vi "Main.vi"(11 "Module Admin":refnum<class "Delacor_lib_QMH_Cloneable Module Admin.lvclass">) -> ()   [LabVIEW 2024, in "CloneableSubpanel.lvlib"]
doc: "This template is based off of the Queued Message Handler design pattern and the Queued Message Handler project template that ships with LabVIEW.\n\nThe main difference is that the queue is private to this module and communication between modules is performed via Broadcast and Request events.\n\nRequest events are wrapped in public API methods and are handled in the Event Handling Loop (EHL) of this VI. Any module can register for Broadcast events sent by this module. The EHL generates messages based on user interface actions.\n\nThe Message Handling Loop (MHL) processes messages generated by the EHL, or by other messages. The messages are string values, so new messages can be added easily to the Message Cases case structure in the MHL. Each message cluster can also provide an optional value for Message Data, which is a variant that can be converted to whatever message-specific data is required.\n_____\nBased on DQMH Dev Tools: Project Template 7.1.0.1503."
uses:
  CloneableSubpanel.lvlib
  <vilib>/Delacor/Delacor QMH/Libraries/Cloneable Module Admin_class/Delacor_lib_QMH_Cloneable Module Admin.lvclass
  C:/Program Files (x86)/National Instruments/LabVIEW 2024/vi.lib/Delacor/Delacor QMH/Libraries/Module Admin_class/Delacor_lib_QMH_Module Admin.lvclass
  Module Data--cluster.ctl
  <vilib>/Delacor/Delacor QMH/Libraries/Message Queue_class/Delacor_lib_QMH_Message Queue.lvclass/Delacor_lib_QMH_Message Queue.ctl
  <vilib>/Delacor/Delacor QMH/Libraries/Cloneable Module Admin_class/Delacor_lib_QMH_Cloneable Module Admin.lvclass/Delacor_lib_QMH_Cloneable Module Admin.ctl
  Stop Argument--cluster.ctl
  <vilib>/Delacor/Delacor QMH/Libraries/Module Admin_class/Delacor_lib_QMH_Module Admin.lvclass/Delacor_lib_QMH_Module Admin.ctl
  Draw FP in Subpanel Argument--cluster.ctl
  Remove From Subpanel Argument--cluster.ctl
  <vilib>/Utility/miscctls.llb/LVPointTypeDef.ctl
  <vilib>/Delacor/Delacor QMH/Libraries/Message Queue_class/Delacor_lib_QMH_Enqueue Message (Single).vi
  <vilib>/Delacor/Delacor QMH/Libraries/Cloneable Module Admin_class/Delacor_lib_QMH_Get Module ID.vi
  <vilib>/Delacor/Delacor QMH/Libraries/Module Admin_class/Delacor_lib_QMH_Get External Launch.vi
  <vilib>/Delacor/Delacor QMH/Libraries/Message Queue_class/Delacor_lib_QMH_Message Queue.lvclass
panel:
  out "error out":errorcluster
  out "Status":string
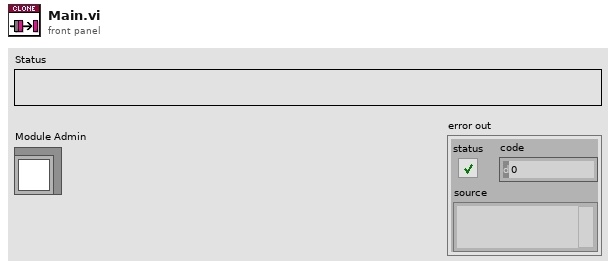
[diagram p1: front panel]
types:
  T1 = typedef "CloneableSubpanel.lvlib/Request Events--cluster.ctl" = cluster{"Stop Module":refnum<user-event>, "Show Panel":refnum<user-event>, "Hide Panel":refnum<user-event>, "Show Diagram":refnum<user-event>, "Get Module Execution Status":refnum<user-event>, "Draw FP in Subpanel":refnum<user-event>, "Remove From Subpanel":refnum<user-event>}
  T2 = typedef "CloneableSubpanel.lvlib/Module Data--cluster.ctl" = cluster{"Status":string, "Sub Panel":refnum<vi>}
  T3 = enum32{"invalid lock state", "Not Locked", "Locked (No Password)", "Password-protected"}
  T4 = typedef "CloneableSubpanel.lvlib/Stop Argument--cluster.ctl" = cluster{"Module ID":i32, "Origin":string, "Exit via Stop Module Req?":bool, "Wait for Module to stop?":bool}
  T5 = typedef "CloneableSubpanel.lvlib/Draw FP in Subpanel Argument--cluster.ctl" = cluster{"Module ID":i32, "Sub Panel":refnum<vi>}
  T6 = typedef "CloneableSubpanel.lvlib/Remove From Subpanel Argument--cluster.ctl" = cluster{"Module ID":i32, "Boolean":bool}
  T7 = typedef "LVPointTypeDef.ctl" = cluster{"Horizontal":i16, "Vertical":i16}
  T8 = enum32{"Invalid", "Standard", "Closed", "Hidden", "Minimized", "Maximized"}
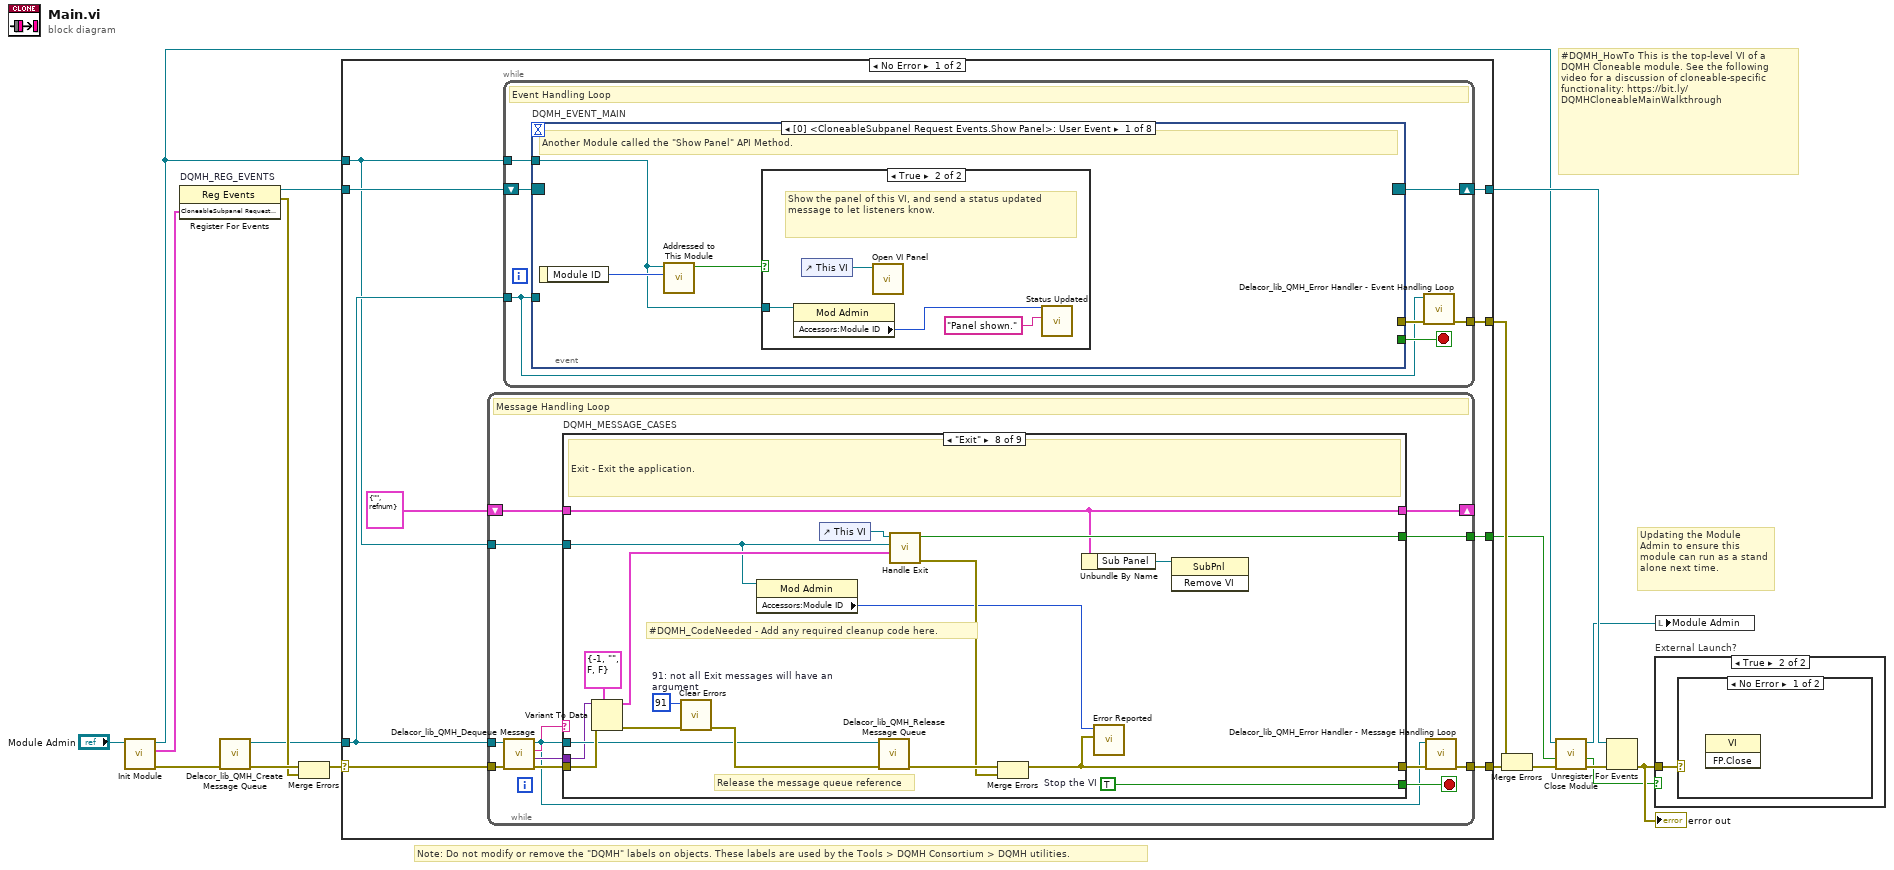
[diagram p0: block diagram]
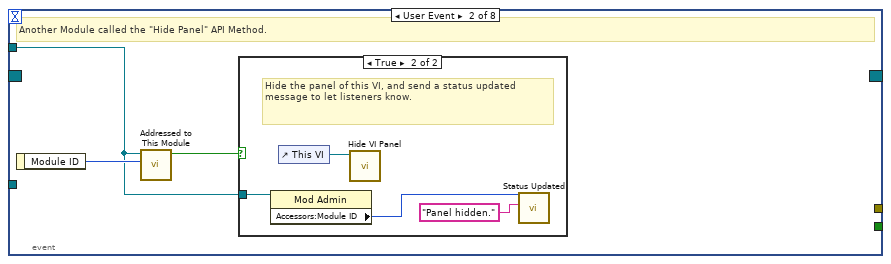
[diagram p3: hidden frame]
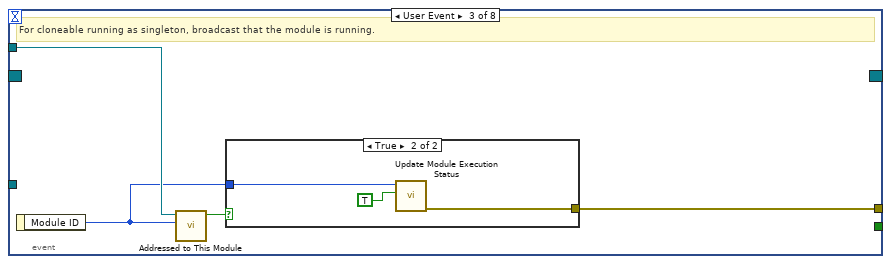
[diagram p5: hidden frame]
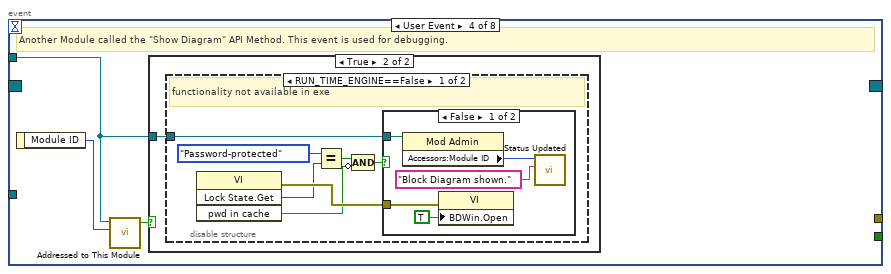
[diagram p7: hidden frame]
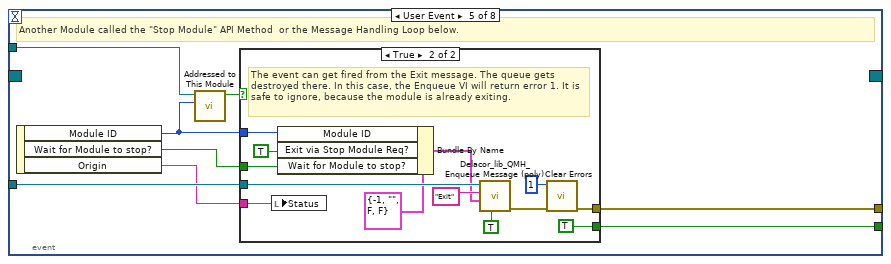
[diagram p11: hidden frame]
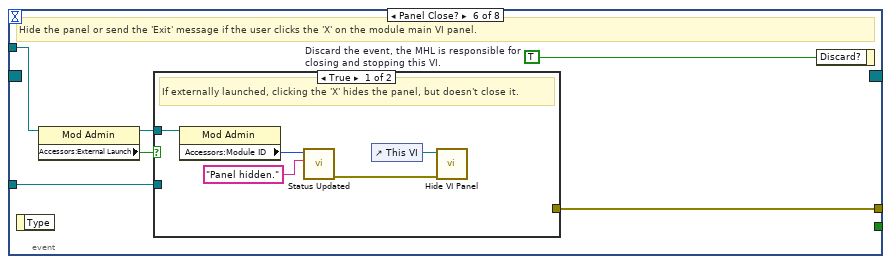
[diagram p13: hidden frame]
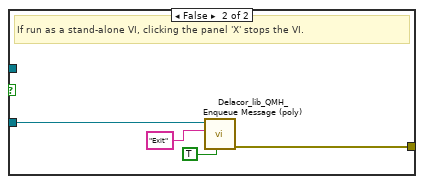
[diagram p14: hidden frame]
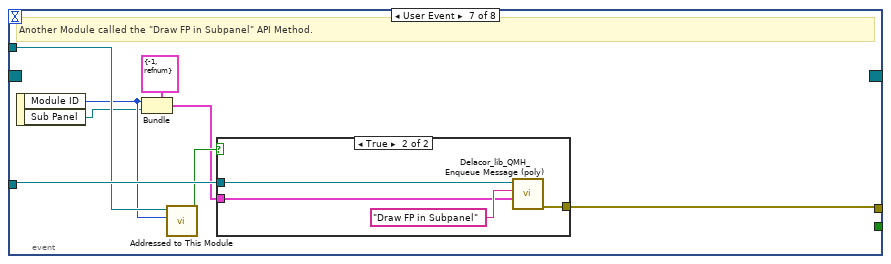
[diagram p15: hidden frame]
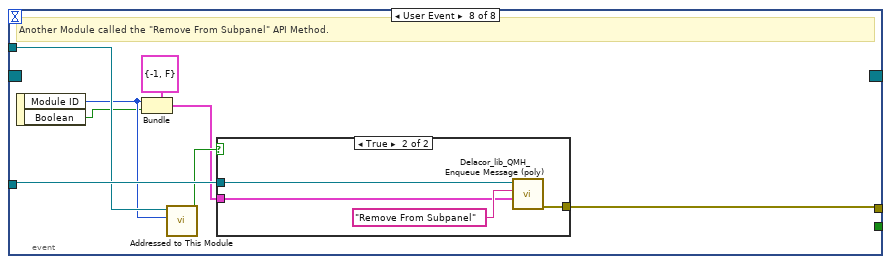
[diagram p17: hidden frame]
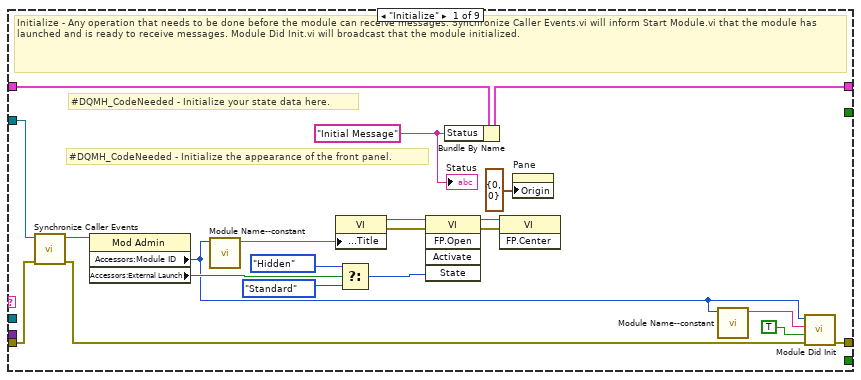
[diagram p19: hidden frame]
diagram:
  # "#DQMH_HowTo This is the top-level VI of a DQMH Cloneable module. See the following video for a discussion of cloneable-specific functionality: https://bit.ly/DQMHCloneableMainWalkthrough"
  # "Note: Do not modify or remove the \"DQMH\" labels on objects. These labels are used by the Tools > DQMH Consortium > DQMH utilities."
  # "Updating the Module Admin to ensure this module can run as a stand alone next time."
  n1 = call "Init Module.vi"("Cloneable Module Admin in"="Module Admin") -> ("error out"=w15:errorcluster, "CloneableSubpanel Request Events"=w7:T1, "Cloneable Module Admin out"=w4:refnum<class "Delacor_lib_QMH_Cloneable Module Admin.lvclass">)  [unwired: 8 in]
  n2 = register-events "DQMH_REG_EVENTS"(w7) -> (reference out=w8:refnum<event-registration>, error out=w10:errorcluster)  [unwired: 2 in]
  n3 = call <vilib>:"Delacor_lib_QMH_Create Message Queue.vi"("error in"=w15) -> ("error out"=w12:errorcluster, "Message Queue"=w6:refnum<class "Delacor_lib_QMH_Message Queue.lvclass">)  [unwired: 9 in]
  n4 = Merge Errors(w12, w10) -> (w11:errorcluster)
  n5 = case shown="No Error" w11 {
    selector: w11 -> [w25 w275]
    tunnel: [w27 w274] -> w16
    tunnel: [w24 w273] -> w9
    tunnel: w8 -> [w22 w273]
    tunnel: w6 -> [w21 w266]
    tunnel: [w26 _] -> w17
    tunnel: w4 -> [w20 w269]
    tunnel: [w19 _] -> w2
    frame No Error {
      n6 = while {
        tunnel: w21 -> [w132]
        shift-right: [w139] -> _
        shift-left: T2 {"Status"="", "Sub Panel"=refnum} ("Data Cluster") -> [w140]
        tunnel: w25 -> [w143]
        tunnel: [w141] -> w27
        tunnel: w20 -> [w134]
        tunnel: [w133] -> w19
        stop <- w138 stop-if-true
        # "Message Handling Loop"
        n7 = call-dynamic "Delacor_lib_QMH_Dequeue Message.vi"("error in"=w143, "Message Queue in"=w132) -> ("error out"=w142:errorcluster, "Message Data"=w136:variant, "Message"=w137:string, "Message Queue out"=w135:refnum<class "Delacor_lib_QMH_Message Queue.lvclass">)  [unwired: 6 in]
        n8 = case "DQMH_MESSAGE_CASES" shown="\"Exit\"" w137 {
          selector: w137 -> [_ _ _ _ _ _ _ _ w255]
          tunnel: w135 -> [_ _ _ _ _ _ w219 w247 _]
          tunnel: w142 -> [w163 w167 w186 w206 w215 w217 w229 w253 w264]
          tunnel: [w161 w167 w182 w204 w214 w217 w225 w248 w265] -> w144
          tunnel: w140 -> [w154 w166 w172 w198 w213 w216 w223 w237 w262]
          tunnel: [w153 w166 w173 w194 w213 w216 w223 w237 w262] -> w139
          tunnel: [_ _ _ _ _ _ _ w246 _] -> w138
          tunnel: w136 -> [_ _ w181 w203 _ _ w222 w244 _]
          tunnel: w134 -> [w149 _ w170 w197 _ _ w221 w239 w261]
          tunnel: [_ _ _ _ _ _ _ w242 _] -> w133
          frame "Initialize" {
            w146 = "Initial Message" ("Initial Message")
            # "#DQMH_CodeNeeded - Initialize the appearance of the front panel."
            # "#DQMH_CodeNeeded - Initialize your state data here."
            # "Initialize - Any operation that needs to be done before the module can receive messages. Synchronize Caller Events.vi will inform Start Module.vi that the module has launched and is ready to receive messages. Module Did Init.vi will broadcast that the module initialized."
            n9 = call "Synchronize Caller Events.vi"("error in"=w163, "Module Admin"=w149) -> ("error out"=w162:errorcluster, "Module Admin out"=w148:refnum<class "Delacor_lib_QMH_Cloneable Module Admin.lvclass">)  [unwired: 8 in]
            n10 = property on="Property Node" class="Mod Admin"(reference=w148) -> ("Accessors:Module ID"=w145:i32, "Accessors:External Launch"=w150:bool)  [unwired: 1 in, 2 out]
            n11 = call "Module Name--constant.vi"("Module ID"=w145) -> ("Module Name"=w158:string)  [unwired: 10 in]
            n12 = property on="Property Node" class="VI"("Front Panel.Title"=w158) -> (reference out=w160:refnum<vi>, error out=w165:errorcluster)  [unwired: 2 in]
            n13 = Select(t=T8."Hidden" ("State"), s=w150, f=T8."Standard" ("State")) -> (s? t:f=w155:T8)
            n14 = invoke on="Invoke Node" class="VI" method="FP.Open"(reference=w160, error in=w165, "State"=w155) -> (reference out=w159:refnum<vi>, error out=w164:errorcluster)  [unwired: 2 in, 3 out]
            n15 = Bundle By Name(cluster=w154, "Status"=w146) -> (w153:T2)
            n16 = invoke on="Invoke Node" class="VI" method="FP.Center"(reference=w159, error in=w164) -> ()  [unwired: 1 in, 3 out]
            n17 = property on="Pane" class="Pane"("Origin"=T7 {"Horizontal"=0, "Vertical"=0}) -> ()  [unwired: 2 in, 2 out]
            n18 = call "Module Name--constant.vi"("Module ID"=w145) -> ("Module Name"=w151:string)  [unwired: 10 in]
            n19 = call "Module Did Init.vi"("error in"=w162, "Initialized?"=TRUE, "Origin"=w151, "Module ID"=w145) -> ("error out"=w161:errorcluster)  [unwired: 7 in]
            "Status" <- w146
          }
          frame "---Module Specific---" {
            # "Separator -- The following cases handle messages specific to this Module."
          }
          frame "Draw FP in Subpanel" {
            # "Draw FP in Subpanel"
            n20 = Variant To Data(error in=w186, type=T5 {"Module ID"=-1, "Sub Panel"=refnum} ("Draw FP in Subpanel Argument"), Variant=w181) -> (data=w179:T5, error out=w183:errorcluster)
            n21 = property class="Mod Admin"(reference=w170) -> ("Accessors:Module ID"=w169:i32)  [unwired: 1 in, 2 out]
            n22 = Unbundle By Name(w179) -> ("Sub Panel"=w171:refnum<vi>)
            n23 = control-ref of="This VI"() -> (w176:refnum<vi>)
            n24 = property class="VI"(reference=w176, error in=w183) -> (reference out=w175:refnum<vi>, error out=w184:errorcluster, "FP.State"=w174:T8)
            n25 = case shown="\"Closed\"" w174 {
              tunnel: [w187 w190] -> w177
              tunnel: [w188 w192] -> w185
              tunnel: w184 -> [w188 w191]
              tunnel: w175 -> [w187 w189]
              frame "Closed" {
              }
              frame "Standard", Default {
                n26 = invoke class="VI" method="FP.Close"(reference=w189, error in=w191) -> (reference out=w190:refnum<vi>, error out=w192:errorcluster)  [unwired: 1 in, 1 out]
              }
            }
            n27 = invoke class="SubPnl" method="Insert VI"(reference=w171, error in=w185, "VI Ref"=w177) -> (reference out=w178:refnum<vi>, error out=w182:errorcluster)  [unwired: 1 in, 2 out]
            n28 = call "Status Updated.vi"("error in"=w182, "Status"="Front Panel Inserted in Subpanel", "Module ID"=w169) -> ()  [unwired: 8 in, 1 out]
            n29 = Bundle By Name(cluster=w172, "Sub Panel"=w178) -> (w173:T2)
          }
          frame "Remove From Subpanel" {
            # "Remove From Subpanel"
            n30 = Variant To Data(error in=w206, type=T6 {"Module ID"=-1, "Boolean"=FALSE} ("Remove From Subpanel Argument"), Variant=w203) -> (data=w201:T6, error out=w205:errorcluster)
            n31 = Unbundle By Name(w201) -> ()  [unwired: 2 out]
            n32 = property class="Mod Admin"(reference=w197) -> ("Accessors:Module ID"=w196:i32)  [unwired: 1 in, 2 out]
            n33 = Unbundle By Name(w198) -> ("Sub Panel"=w200:refnum<vi>)
            n34 = Not A Number/Path/Refnum?(number/path/refnum=w200) -> (NaN/Path/Refnum?=w199:bool)
            n35 = case shown="False" w199 {
              tunnel: w205 -> [w210 w212]
              tunnel: [w209 w212] -> w204
              tunnel: w200 -> [w208 _]
              tunnel: ["Panel Removed from Subpanel" "This module has not been inserted into the subpanel"] -> w195
              frame False {
                n36 = invoke class="SubPnl" method="Remove VI"(reference=w208, error in=w210) -> (error out=w209:errorcluster)  [unwired: 1 in, 2 out]
              }
              frame True {
              }
            }
            n37 = Bundle By Name(cluster=w198, "Sub Panel"=refnum<vi> refnum) -> (w194:T2)
            n38 = call "Status Updated.vi"("error in"=w204, "Status"=w195, "Module ID"=w196) -> ()  [unwired: 8 in, 1 out]
          }
          frame "---Copy This Frame---" {
            # "Duplicate this frame when creating new messages.  Change this comment in the duplicated frame to describe this message."
            n39 = Merge Errors(w215) -> (w214:errorcluster)
          }
          frame "---Exit and Error Handling---" {
            # "Separator - the following cases handle errors and exit messages."
          }
          frame "Error" {
            # "#DQMH_CodeRecommended - If the module is running in standalone mode (External Launch = FALSE), this code will pop up an error dialog and call the 'Exit' message if an error occurs. Add more fine-grained error management here."
            # "Error - Check the error message data and respond accordingly. This message is sent by the \"Error Handler\" VIs at the end of each loop in this application."
            n40 = property on="Property Node" class="Mod Admin"(reference=w221) -> ("Accessors:External Launch"=w220:bool, "Accessors:Module ID"=w218:i32)  [unwired: 1 in, 2 out]
            n41 = Variant To Data(error in=w229, type=errorcluster {"status"=FALSE, "code"=0, "source"=""} ("error constant"), Variant=w222) -> (data=w224:errorcluster, error out=w227:errorcluster)
            n42 = local write "error out"(w224) -> ()
            n43 = call "Error Reported.vi"("Error"=w224, "Module ID"=w218) -> ()  [unwired: 9 in, 1 out]
            n44 = case shown="False" w220 {
              tunnel: [w234 _] -> w226
              tunnel: w219 -> [w232 _]
              tunnel: w224 -> [w233 _]
              frame False {
                n45 = disable-structure shown="Default" {
                  disable-tunnel: w233 -> [w235 _]
                  frame condition #0 (active) {
                    # "If the module is running standalone, then pop up an error dialog and call the \"Exit\" message."
                    n46 = call <vilib>:"Simple Error Handler.vi"("error in (no error)"=w235) -> ()  [unwired: 4 in, 5 out]
                  }
                  frame condition #1 {
                    # "To prevent the Simple Error Handler VI from being loaded (e.g. when deploying to a Real-Time target), add the Conditional Disable Symbol \"DQMH_Disable_SEH\" to your project and set it to TRUE."
                  }
                }
                n47 = call-poly <vilib>:"Delacor_lib_QMH_Enqueue Message (poly).vi"("Priority Message? (F)"=TRUE, "Message"="Exit", "Message Queue in"=w232) -> ("error out"=w234:errorcluster)  [unwired: 7 in, 1 out]
              }
              frame True {
                # "If the module was launched externally, calling the Error Reported broadcast VI is the only action performed by the \"Error\" message. The module's caller can then process the error appropriately."
              }
            }
            n48 = Merge Errors(w227, w226) -> (w225:errorcluster)
          }
          frame "Exit" {
            w245 = 91  # 91: not all Exit messages will have an argument
            w246 = TRUE  # Stop the VI
            # "Release the message queue reference"
            # "#DQMH_CodeNeeded - Add any required cleanup code here."
            # "Exit - Exit the application."
            n49 = Variant To Data(error in=w253, type=T4 {"Module ID"=-1, "Origin"="", "Exit via Stop Module Req?"=FALSE, "Wait for Module to stop?"=FALSE} ("Stop Argument"), Variant=w244) -> (data=w241:T4, error out=w249:errorcluster)
            n50 = call <vilib>:"Clear Errors.vi"("error in (no error)"=w249, "specific error code to clear (0: all)"=w245) -> ("error out"=w252:errorcluster)  [unwired: 4 in, 1 out]
            n51 = property on="Property Node" class="Mod Admin"(reference=w239) -> ("Accessors:Module ID"=w238:i32)  [unwired: 1 in, 2 out]
            n52 = control-ref of="This VI"() -> (w240:refnum<vi>)
            n53 = call-dynamic "Delacor_lib_QMH_Release Message Queue.vi"("error in"=w252, "Message Queue"=w247) -> ("error out"=w251:errorcluster)  [unwired: 9 in]
            n54 = call "Handle Exit.vi"("Stop Argument"=w241, "Module Admin in"=w239, "VI reference"=w240) -> ("error out"=w250:errorcluster, "Wait for Stop?"=w242:bool)  [unwired: 7 in]
            n55 = Merge Errors(w251, w250) -> (w248:errorcluster)
            n56 = Unbundle By Name(w237) -> ("Sub Panel"=w236:refnum<vi>)
            n57 = call "Error Reported.vi"("Error"=w248, "Module ID"=w238) -> ()  [unwired: 9 in, 1 out]
            n58 = invoke class="SubPnl" method="Remove VI"(reference=w236) -> ()  [unwired: 2 in, 3 out]
          }
          frame Default {
            # "'Default' case only runs if there is a message that isn't defined in any of the other cases.  Output a programming error."
            n59 = property on="Property Node" class="Mod Admin"(reference=w261) -> ("Accessors:Module ID"=w260:i32)  [unwired: 1 in, 2 out]
            n60 = call "Module Name--constant.vi"("Module ID"=w260) -> ("Module Name"=w254:string)  [unwired: 10 in]
            n61 = Format Into String(format string="The invalid message string \"%s\" was received in the Message Handling Loop for module \"%s\".", w255, w254) -> (resulting string=w257:string)  [unwired: 2 in, 1 out]
            n62 = call <vilib>:"Error Cluster From Error Code.vi"("show call chain? (False)"=TRUE, "error message (\"\")"=w257, "error code (0)"=1) -> ("error out"=w263:errorcluster)  [unwired: 6 in]
            n63 = Merge Errors(w264, w263) -> (w265:errorcluster)
          }
        }
        n64 = call-dynamic "Delacor_lib_QMH_Error Handler - Message Handling Loop.vi"("error in"=w144, "Message Queue in"=w135) -> ("dup error in"=w141:errorcluster)  [unwired: 8 in, 1 out]
      }
      n65 = while {
        tunnel: w21 -> [w28]
        shift-right: [w31] -> w24
        shift-left: w22 -> [w32]
        tunnel: [w33] -> w26
        tunnel: w20 -> [w29]
        stop <- w30 stop-if-true
        # "Event Handling Loop"
        n66 = event "DQMH_EVENT_MAIN" shown="[0] <CloneableSubpanel Request Events.Show Panel>: User Event" {
          selector: w32 -> [_ _ _ _ _ _ _ _]
          dyn-events: [_ _ _ _ _ _ _ _] -> w31
          timeout: _ -> [_ _ _ _ _ _ _ _]
          tunnel: [_ _ _ _ w75 _ _ _] -> w30
          tunnel: w28 -> [_ _ _ _ w78 w95 w114 w126]
          tunnel: [_ _ w52 _ w79 w98 w115 w127] -> w34
          tunnel: w29 -> [w35 w42 w50 w56 w77 w96 w112 w124]
          event User Event {
            # "Another Module called the \"Show Panel\" API Method."
            n67 = event-data() -> ("Module ID"=w36:i32)  [unwired: 1 in]
            n68 = call "Addressed to This Module.vi"("Module ID from Argument"=w36, "Module Admin"=w35) -> ("Addressed to this instance?"=w37:bool)  [unwired: 8 in, 1 out]
            n69 = case shown="True" w37 {
              tunnel: w35 -> [_ w39]
              frame False {
              }
              frame True {
                # "Show the panel of this VI, and send a status updated message to let listeners know."
                n70 = property on="Property Node" class="Mod Admin"(reference=w39) -> ("Accessors:Module ID"=w38:i32)  [unwired: 1 in, 2 out]
                n71 = control-ref of="This VI"() -> (w41:refnum<vi>)
                n72 = call "Open VI Panel.vi"("VI"=w41) -> ()  [unwired: 10 in, 1 out]
                n73 = call "Status Updated.vi"("Status"="Panel shown." ("format string"), "Module ID"=w38) -> ()  [unwired: 9 in, 1 out]
              }
            }
          }
          event User Event {
            # "Another Module called the \"Hide Panel\" API Method."
            n74 = event-data() -> ("Module ID"=w43:i32)  [unwired: 1 in]
            n75 = call "Addressed to This Module.vi"("Module ID from Argument"=w43, "Module Admin"=w42) -> ("Addressed to this instance?"=w44:bool)  [unwired: 8 in, 1 out]
            n76 = case shown="True" w44 {
              tunnel: w42 -> [_ w46]
              frame False {
              }
              frame True {
                # "Hide the panel of this VI, and send a status updated message to let listeners know."
                n77 = property on="Property Node" class="Mod Admin"(reference=w46) -> ("Accessors:Module ID"=w45:i32)  [unwired: 1 in, 2 out]
                n78 = control-ref of="This VI"() -> (w48:refnum<vi>)
                n79 = call "Hide VI Panel.vi"("VI"=w48) -> ()  [unwired: 10 in, 1 out]
                n80 = call "Status Updated.vi"("Status"="Panel hidden." ("format string"), "Module ID"=w45) -> ()  [unwired: 9 in, 1 out]
              }
            }
          }
          event User Event {
            # "For cloneable running as singleton, broadcast that the module is running."
            n81 = event-data() -> ("Module ID"=w49:i32)  [unwired: 1 in]
            n82 = call "Addressed to This Module.vi"("Module ID from Argument"=w49, "Module Admin"=w50) -> ("Addressed to this instance?"=w51:bool)  [unwired: 8 in, 1 out]
            n83 = case shown="True" w51 {
              tunnel: [_ w55] -> w52
              tunnel: w49 -> [_ w54]
              frame False {
              }
              frame True {
                n84 = call "Update Module Execution Status.vi"("Running?"=TRUE, "Module ID"=w54) -> ("error out"=w55:errorcluster)  [unwired: 9 in]
              }
            }
          }
          event User Event {
            # "Another Module called the \"Show Diagram\" API Method. This event is used for debugging."
            n85 = event-data() -> ("Module ID"=w57:i32)  [unwired: 1 in]
            n86 = call "Addressed to This Module.vi"("Module ID from Argument"=w57, "Module Admin"=w56) -> ("Addressed to this instance?"=w58:bool)  [unwired: 8 in, 1 out]
            n87 = case shown="True" w58 {
              tunnel: w56 -> [_ w59]
              frame False {
              }
              frame True {
                n88 = disable-structure shown="RUN_TIME_ENGINE==False" {
                  disable-tunnel: w59 -> [w60 _]
                  frame condition #0 (active) {
                    # "functionality not available in exe"
                    n89 = invoke on="Invoke Node" class="VI" method="Lock State.Get"() -> (error out=w66:errorcluster, "Get Lock State"=w65:T3, "pwd in cache"=w62:bool)  [unwired: 4 in, 1 out]
                    n90 = Equal?(x=T3."Password-protected", y=w65) -> (x = y?=w63:bool)
                    n91 = Compound Arithmetic op=AND(w63, invert w62) -> (w61:bool)
                    n92 = case shown="False" w61 {
                      tunnel: w66 -> [w71 _]
                      tunnel: w60 -> [w68 _]
                      frame False {
                        n93 = property on="Property Node" class="Mod Admin"(reference=w68) -> ("Accessors:Module ID"=w67:i32)  [unwired: 1 in, 2 out]
                        n94 = property on="Property Node" class="VI"(error in=w71, "BDWin.Open"=TRUE ("Block Diagram Window:Open")) -> ()  [unwired: 1 in, 2 out]
                        n95 = call "Status Updated.vi"("Status"="Block Diagram shown." ("format string"), "Module ID"=w67) -> ()  [unwired: 9 in, 1 out]
                      }
                      frame True {
                        # "Password-protected VI, and the password is not in the cache. Do not show the diagram."
                      }
                    }
                  }
                  frame condition #1 {
                  }
                }
              }
            }
          }
          event User Event {
            # "Another Module called the \"Stop Module\" API Method  or the Message Handling Loop below."
            n96 = event-data() -> ("Module ID"=w73:i32, "Wait for Module to stop?"=w74:bool, "Origin"=w72:string)  [unwired: 1 in]
            n97 = call "Addressed to This Module.vi"("Module ID from Argument"=w73, "Module Admin"=w77) -> ("Addressed to this instance?"=w76:bool)  [unwired: 8 in, 1 out]
            n98 = case shown="True" w76 {
              tunnel: [_ w91] -> w79
              tunnel: w78 -> [_ w87]
              tunnel: [_ TRUE] -> w75
              tunnel: w74 -> [_ w82]
              tunnel: w73 -> [_ w84]
              tunnel: w72 -> [_ w80]
              frame False {
              }
              frame True {
                # "The event can get fired from the Exit message. The queue gets destroyed there. In this case, the Enqueue VI will return error 1. It is safe to ignore, because the module is already exiting."
                n99 = local write "Status"(w80) -> ()
                n100 = Bundle By Name(cluster=T4 {"Module ID"=-1, "Origin"="", "Exit via Stop Module Req?"=FALSE, "Wait for Module to stop?"=FALSE} ("Stop Argument"), "Module ID"=w84, "Exit via Stop Module Req?"=TRUE, "Wait for Module to stop?"=w82) -> (w81:T4)
                n101 = call-poly <vilib>:"Delacor_lib_QMH_Enqueue Message (poly).vi"("Priority Message? (F)"=TRUE, "Message Data"=w81, "Message"="Exit", "Message Queue in"=w87) -> ("error out"=w92:errorcluster)  [unwired: 6 in, 1 out]
                n102 = call <vilib>:"Clear Errors.vi"("error in (no error)"=w92, "specific error code to clear (0: all)"=1) -> ("error out"=w91:errorcluster)  [unwired: 4 in, 1 out]
              }
            }
          }
          event Panel Close? {
            w97 = TRUE  # Discard the event, the MHL is responsible for closing and stopping this VI.
            # "Hide the panel or send the 'Exit' message if the user clicks the 'X' on the module main VI panel."
            n103 = event-data() -> ()  [unwired: 1 in, 1 out]
            n104 = property on="Property Node" class="Mod Admin"(reference=w96) -> (reference out=w93:refnum<class "Delacor_lib_QMH_Cloneable Module Admin.lvclass">, "Accessors:External Launch"=w94:bool)  [unwired: 1 in, 1 out]
            n105 = case shown="True" w94 {
              tunnel: w95 -> [_ w106]
              tunnel: [_ w107] -> w98
              tunnel: w93 -> [w100 _]
              frame True {
                # "If externally launched, clicking the 'X' hides the panel, but doesn't close it."
                n106 = property on="Property Node" class="Mod Admin"(reference=w100) -> ("Accessors:Module ID"=w99:i32)  [unwired: 1 in, 2 out]
                n107 = call "Status Updated.vi"("Status"="Panel hidden." ("format string"), "Module ID"=w99) -> ("error out"=w103:errorcluster)  [unwired: 9 in]
                n108 = control-ref of="This VI"() -> (w102:refnum<vi>)
                n109 = call "Hide VI Panel.vi"("error in"=w103, "VI"=w102) -> ()  [unwired: 9 in, 1 out]
              }
              frame False {
                # "If run as a stand-alone VI, clicking the panel 'X' stops the VI."
                n110 = call-poly <vilib>:"Delacor_lib_QMH_Enqueue Message (poly).vi"("Priority Message? (F)"=TRUE, "Message"="Exit", "Message Queue in"=w106) -> ("error out"=w107:errorcluster)  [unwired: 7 in, 1 out]
              }
            }
            n111 = event-data ("Event Filter Node")("Discard?"=w97) -> ()  [unwired: 1 in, 1 out]
          }
          event User Event {
            # "Another Module called the \"Draw FP in Subpanel\" API Method."
            n112 = event-data() -> ("Module ID"=w109:i32, "Sub Panel"=w108:refnum<vi>)  [unwired: 1 in]
            n113 = Bundle(cluster=T5 {"Module ID"=-1, "Sub Panel"=refnum} ("Draw FP in Subpanel Argument"), "Module ID"=w109, "Sub Panel"=w108) -> (w110:T5)
            n114 = call "Addressed to This Module.vi"("Module ID from Argument"=w109, "Module Admin"=w112) -> ("Addressed to this instance?"=w113:bool)  [unwired: 8 in, 1 out]
            n115 = case shown="True" w113 {
              tunnel: w114 -> [_ w118]
              tunnel: w110 -> [_ w116]
              tunnel: [_ w119] -> w115
              frame False {
              }
              frame True {
                n116 = call-poly <vilib>:"Delacor_lib_QMH_Enqueue Message (poly).vi"("Message Data"=w116, "Message"="Draw FP in Subpanel", "Message Queue in"=w118) -> ("error out"=w119:errorcluster)  [unwired: 7 in, 1 out]
              }
            }
          }
          event User Event {
            # "Another Module called the \"Remove From Subpanel\" API Method."
            n117 = event-data() -> ("Module ID"=w121:i32, "Boolean"=w120:bool)  [unwired: 1 in]
            n118 = Bundle(cluster=T6 {"Module ID"=-1, "Boolean"=FALSE} ("Remove From Subpanel Argument"), "Module ID"=w121, "Boolean"=w120) -> (w122:T6)
            n119 = call "Addressed to This Module.vi"("Module ID from Argument"=w121, "Module Admin"=w124) -> ("Addressed to this instance?"=w125:bool)  [unwired: 8 in, 1 out]
            n120 = case shown="True" w125 {
              tunnel: w126 -> [_ w130]
              tunnel: w122 -> [_ w128]
              tunnel: [_ w131] -> w127
              frame False {
              }
              frame True {
                n121 = call-poly <vilib>:"Delacor_lib_QMH_Enqueue Message (poly).vi"("Message Data"=w128, "Message"="Remove From Subpanel", "Message Queue in"=w130) -> ("error out"=w131:errorcluster)  [unwired: 7 in, 1 out]
              }
            }
          }
        }
        n122 = call-dynamic "Delacor_lib_QMH_Error Handler - Event Handling Loop.vi"("error in"=w34, "Message Queue in"=w28) -> ("dup error in"=w33:errorcluster)  [unwired: 8 in, 1 out]
      }
    }
    frame Error {
      n123 = call "Synchronize Caller Events.vi"("Module Admin"=w269) -> ("Module Admin out"=w268:refnum<class "Delacor_lib_QMH_Cloneable Module Admin.lvclass">)  [unwired: 9 in, 1 out]
      n124 = property on="Property Node" class="Mod Admin"(reference=w268) -> ("Accessors:Module ID"=w267:i32)  [unwired: 1 in, 2 out]
      n125 = call-dynamic "Delacor_lib_QMH_Release Message Queue.vi"("error in"=w275, "Message Queue"=w266) -> ("error out"=w274:errorcluster)  [unwired: 9 in]
      n126 = call "Module Name--constant.vi"("Module ID"=w267) -> ("Module Name"=w272:string)  [unwired: 10 in]
      n127 = Format Into String(format string="An error occurred during initialization. %s is no longer running.", w272) -> (resulting string=w270:string)  [unwired: 2 in, 1 out]
      n128 = call "Error Reported.vi"("Additional Information"=w270, "Error"=w274, "Module ID"=w267) -> ()  [unwired: 8 in, 1 out]
    }
  }
  n129 = Merge Errors(w17, w16) -> (w18:errorcluster)
  n130 = call "Close Module.vi"("error in"=w18, "Wait for stop?"=w2, "Module Admin in"=w4) -> ("error out"=w14:errorcluster, "External Launch"=w1:bool, "Module Admin out"=w3:refnum<class "Delacor_lib_QMH_Cloneable Module Admin.lvclass">)  [unwired: 6 in]
  n131 = Unregister For Events(event registration refnum=w9, error in=w14) -> (error out=w13:errorcluster)
  "error out" <- w13
  n132 = case "External Launch?" shown="True" w1 {
    tunnel: w13 -> [_ w276]
    frame False {
    }
    frame True {
      n133 = case shown="No Error" w276 {
        frame No Error {
          n134 = invoke class="VI" method="FP.Close"() -> ()  [unwired: 3 in, 3 out]
        }
        frame Error {
          n135 = disable-structure shown="Default" {
            frame condition #0 (active) {
              n136 = invoke class="VI" method="FP.Open"("Activate"=TRUE ("Activate?")) -> ()  [unwired: 4 in, 5 out]
            }
            frame condition #1 {
              # "Don't show panel on error if running inside a built EXE."
            }
          }
        }
      }
    }
  }
  n137 = local write "Module Admin"(w3) -> ()
